vi "Save_Points(X-Y)_Areas-2.vi"(3 "error IN":errorcluster, 5 "[IN] Cluster of \npoints and areas":T1(array[cluster])) -> (0 "error OUT":errorcluster, 1 "[OUT] Areas":dbl[][](array[numeric]), 2 "[OUT] Points (X,Y)":dbl[][](array[numeric]))   [LabVIEW 2017]
doc: "SubVI resaves dots from clusters to big 2D array (old data types, but many other functions demands it)"
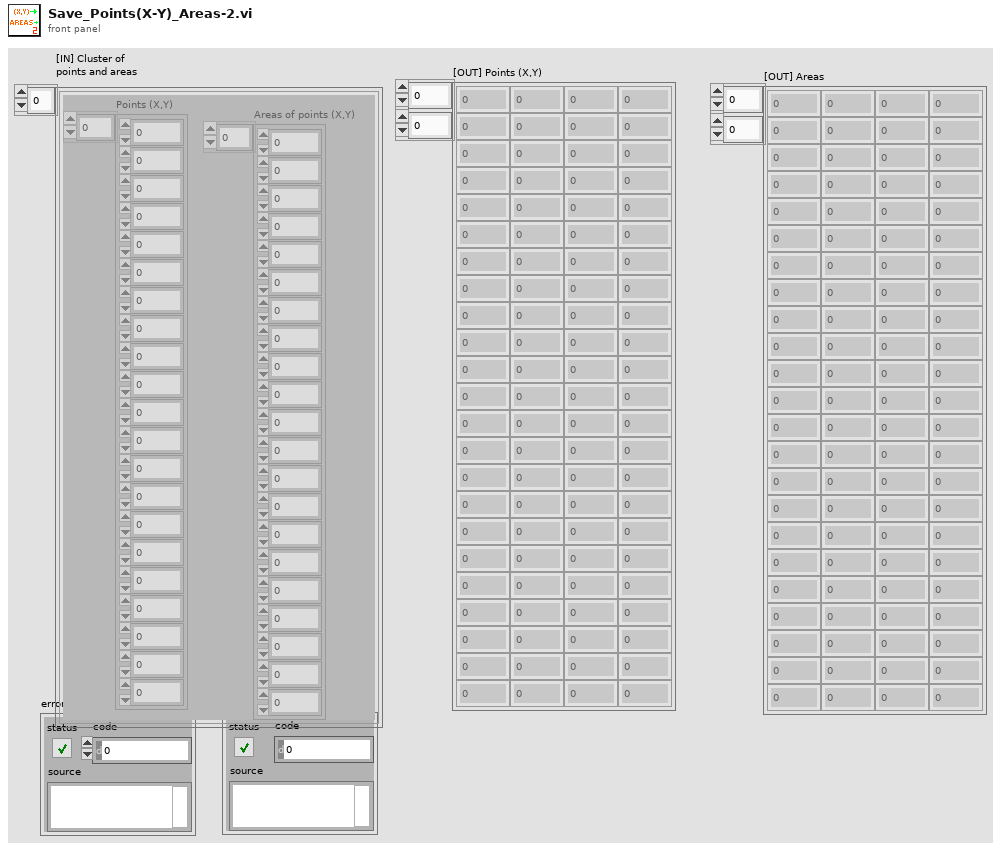
[diagram p1: front panel]
types:
  T1 = cluster{"Points (X,Y)":dbl[], "Areas of points (X,Y)":dbl[]}[]
  T2 = cluster{"Points (X,Y)":dbl[], "Areas of points (X,Y)":dbl[]}
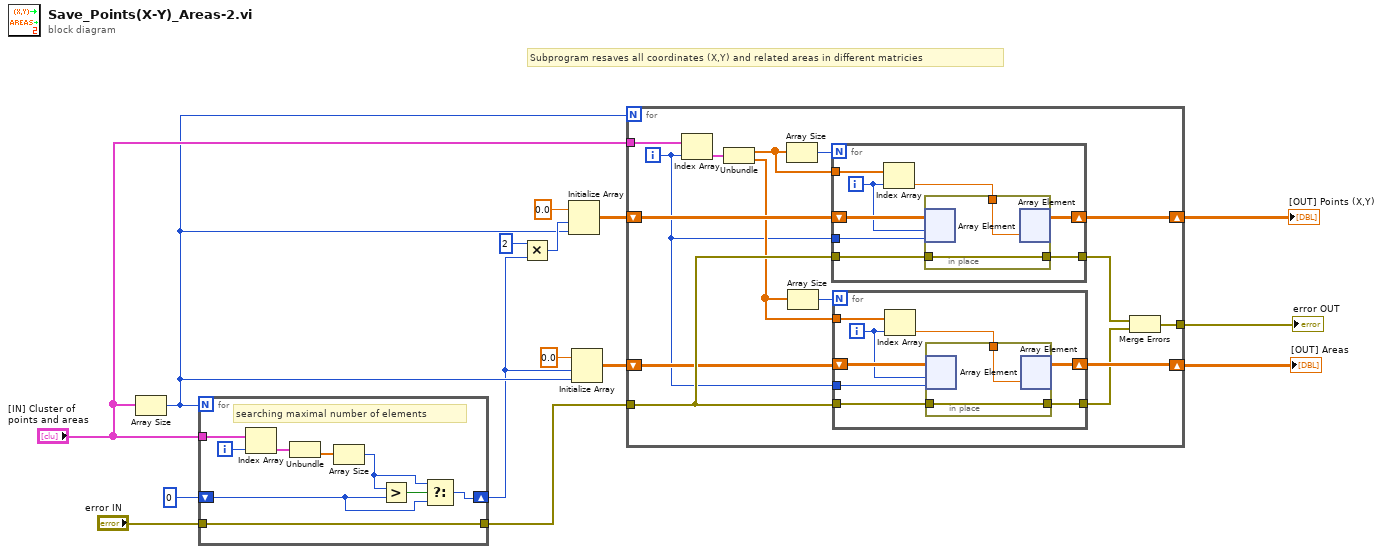
[diagram p0: block diagram]
diagram:
  # "Subprogram resaves all coordinates (X,Y) and related areas in different matricies"
  n1 = Array Size(array="[IN] Cluster of \npoints and areas") -> (size(s)=w7:i32)
  n2 = for {
    N: w7 -> [_]
    tunnel: "[IN] Cluster of \npoints and areas" -> [w24]
    shift-right: [w19] -> w5
    shift-left: 0 -> [w16]
    tunnel: "error IN" -> [w18]
    tunnel: [w18] -> w4
    i -> [w23]
    # "searching maximal number of elements"
    n3 = Index Array(array=w24, index=w23) -> (element=w22:T2)
    n4 = Unbundle(w22) -> ("Areas of points (X,Y)"=w21:dbl[])  [unwired: 1 out]
    n5 = Array Size(array=w21) -> (size(s)=w17:i32)
    n6 = Greater?(x=w17, y=w16) -> (0:w20:bool)
    n7 = Select(t=w17, s=w20, f=w16) -> (s? t:f=w19:i32)
  }
  n8 = Multiply(x=2, y=w5) -> (x*y=w11:i32)
  n9 = Initialize Array(0.0 ("element"), w11, w7) -> (w9:dbl[][])
  n10 = Initialize Array(0.0 ("element"), w5, w7) -> (w6:dbl[][])
  n11 = for {
    N: w7 -> [_]
    tunnel: "[IN] Cluster of \npoints and areas" -> [w39]
    shift-right: [w34] -> w2
    shift-left: w9 -> [w35]
    shift-right: [w29] -> w1
    shift-left: w6 -> [w31]
    tunnel: w4 -> [w32]
    tunnel: [w27] -> w3
    i -> [w25]
    n12 = Index Array(array=w39, index=w25) -> (element=w38:T2)
    n13 = Unbundle(w38) -> ("Points (X,Y)"=w36:dbl[], "Areas of points (X,Y)"=w30:dbl[])
    n14 = Array Size(array=w36) -> (size(s)=w37:i32)
    n15 = Array Size(array=w30) -> (size(s)=w33:i32)
    n16 = for {
      N: w37 -> [_]
      tunnel: w36 -> [w57]
      shift-right: [w52] -> w34
      shift-left: w35 -> [w56]
      tunnel: w25 -> [w54]
      tunnel: w32 -> [w51]
      tunnel: [w50] -> w26
      i -> [w55]
      n17 = Index Array(array=w57, index=w55) -> (element=w53:dbl)
      n18 = in-place {
        in-place-border: w53 -> [w59]
        in-place-border: w51 -> [w58]
        in-place-border: [w58] -> w50
        n19 = in-place-array #1(w56, w55, w54) -> ()  [unwired: 1 out]
        n20 = in-place-array #1(w59) -> (w52:dbl[][])  [unwired: 2 out]
      }
    }
    n21 = for {
      N: w33 -> [_]
      tunnel: w30 -> [w47]
      shift-right: [w42] -> w29
      shift-left: w31 -> [w46]
      tunnel: w25 -> [w44]
      tunnel: w32 -> [w41]
      tunnel: [w40] -> w28
      i -> [w45]
      n22 = Index Array(array=w47, index=w45) -> (element=w43:dbl)
      n23 = in-place {
        in-place-border: w43 -> [w49]
        in-place-border: w41 -> [w48]
        in-place-border: [w48] -> w40
        n24 = in-place-array #2(w46, w45, w44) -> ()  [unwired: 1 out]
        n25 = in-place-array #2(w49) -> (w42:dbl[][])  [unwired: 2 out]
      }
    }
    n26 = Merge Errors(w26, w28) -> (w27:errorcluster)
  }
  "error OUT" <- w3
  "[OUT] Points (X,Y)" <- w2
  "[OUT] Areas" <- w1
